vi "Get All Attributes.vi"(8 "error in (no error)":errorcluster, 11 "Variant in":refnum<class "Variant.lvclass">) -> (0 "error out":errorcluster, 1 "Data":refnum<class "Data.lvclass">[](array[class]), 2 "Names":string[](array[string]), 3 "Variant out":refnum<class "Variant.lvclass">)   [LabVIEW 2020, in "Data.lvlib" / "Variant.lvclass"]
doc: "Get all attributes from the variant."
uses:
  Variant.lvclass
  Data.lvclass
  Variant.lvclass/Variant.ctl
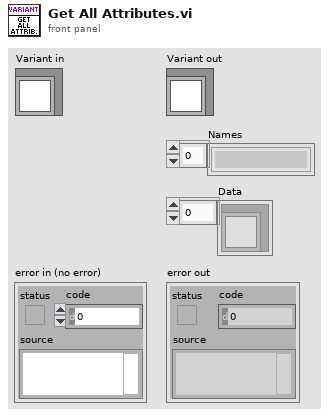
[diagram p1: front panel]
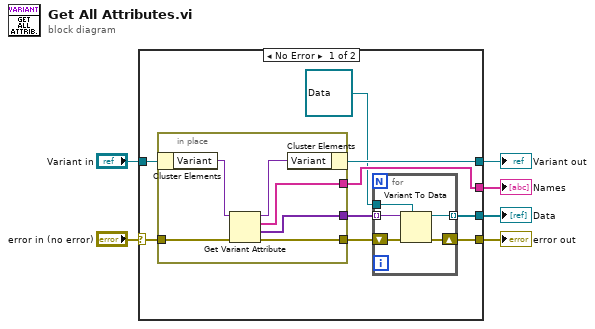
[diagram p0: block diagram]
diagram:
  n1 = case shown="No Error" "error in (no error)" {
    selector: "error in (no error)" -> [w13 w28]
    tunnel: [w7 w28] -> w4
    tunnel: [w14 w27] -> w3
    tunnel: "Variant in" -> [w15 w27]
    tunnel: [w12 _] -> w2
    tunnel: [w9 _] -> w1
    frame No Error {
      n2 = in-place {
        in-place-border: w13 -> [w24]
        in-place-border: [w23] -> w8
        in-place-border: [w22] -> w12
        in-place-border: [w21] -> w11
        n3 = in-place-cluster #1(w15) -> ("Variant"=w26:variant)
        n4 = Get Variant Attribute(Variant=w26, error in=w24) -> (duplicate Variant=w25:variant, names=w22:string[], values=w21:variant[], error out=w23:errorcluster)  [unwired: 2 in]
        n5 = in-place-cluster #1("Variant"=w25) -> (w14:refnum<class "Variant.lvclass">)
      }
      n6 = for {
        tunnel: w11 -> [w20] mode=indexing
        tunnel: refnum<class "Data.lvclass"> refnum ("Data") -> [w19]
        tunnel: [w18] -> w9 mode=indexing
        shift-right: [w16] -> w7
        shift-left: w8 -> [w17]
        n7 = Variant To Data(error in=w17, type=w19, Variant=w20) -> (data=w18:refnum<class "Data.lvclass">, error out=w16:errorcluster)
      }
    }
    frame Error {
    }
  }
  "error out" <- w4
  "Variant out" <- w3
  "Data" <- w1
  "Names" <- w2
